vi "HW_6p1_Task1_weesesr.vi"() -> ()   [LabVIEW 2016]
uses:
  <vilib>/express/express arith-compare/Formula/XNode/ExpressFormulaBlockNode.xnode
panel:
  in  "Target Concentration for C (in mol/L)":dbl
  out "Time passed (in min)":dbl
  out "Concentration C":dbl
  out "Concentration B":dbl
  out "Concentration A":dbl
  in  "K3 (in mol^4/min)":dbl
  in  "K2 (in L / mol*min)":dbl
  in  "K1 (in L^2 / mol^2 *min)":dbl
  in  "B Initial Concentration":dbl
  in  "A Initial Concentration":dbl
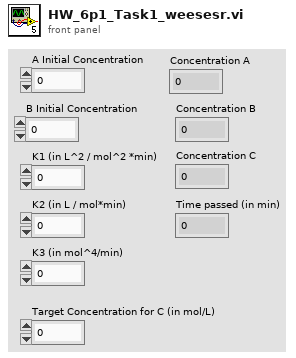
[diagram p1: front panel]
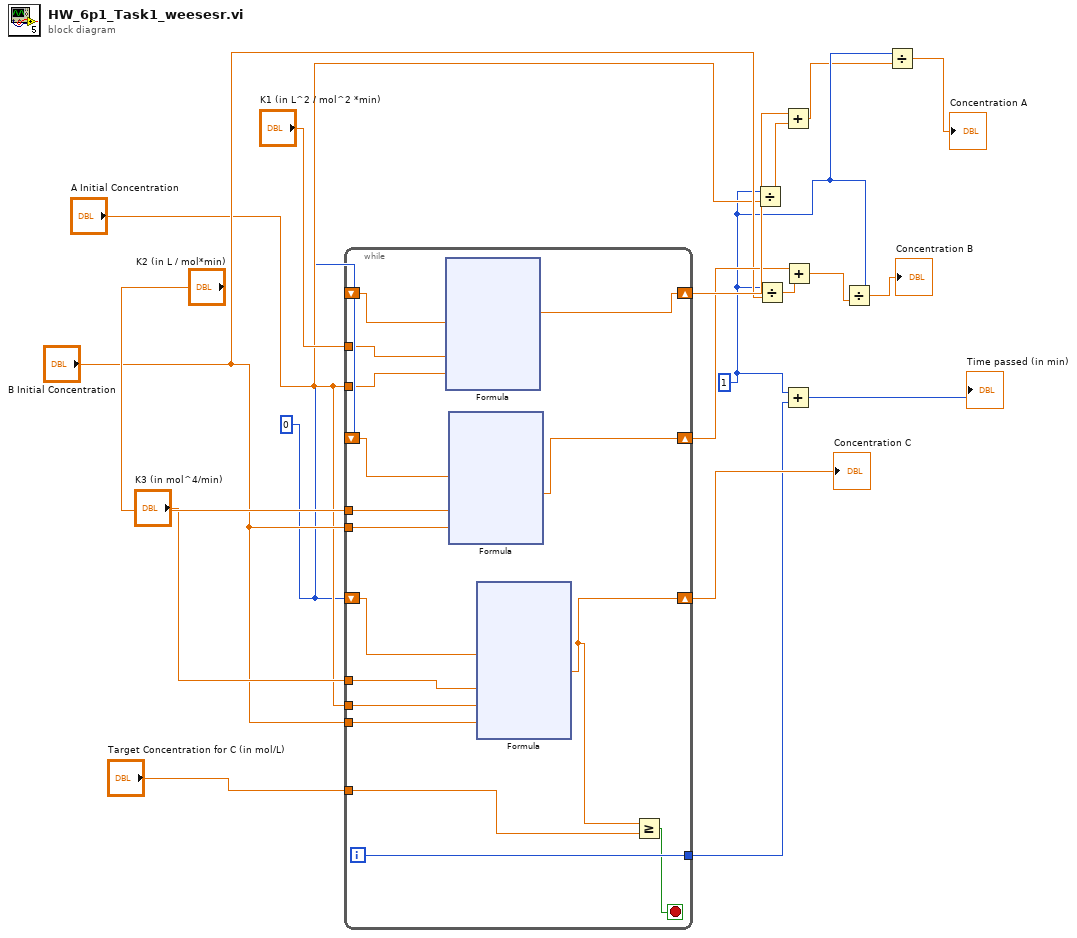
[diagram p0: block diagram]
diagram:
  w8 = 0
  w5 = 1
  n1 = while {
    shift-right: [w20] -> w12
    shift-left: w8 -> [w21]
    tunnel: [w35] -> w7
    shift-right: [w29] -> w11
    shift-left: w8 -> [w30]
    shift-right: [w31] -> w14
    shift-left: w8 -> [w32]
    tunnel: "A Initial Concentration" -> [w34]
    tunnel: "K1 (in L^2 / mol^2 *min)" -> [w33]
    tunnel: "B Initial Concentration" -> [w28]
    tunnel: "K2 (in L / mol*min)" -> [w27]
    tunnel: "K3 (in mol^4/min)" -> [w26]
    tunnel: "Target Concentration for C (in mol/L)" -> [w25]
    tunnel: "B Initial Concentration" -> [w22]
    tunnel: "A Initial Concentration" -> [w23]
    i -> [w35]
    stop <- w24 stop-if-true
    n2 = xnode "Formula"("X1"=w32, "X2"=w33, "X3"=w34) -> ("Result"=w31:dbl)  [unwired: 1 in, 1 out]
    n3 = xnode "Formula"("X1"=w30, "X2"=w27, "X3"=w28) -> ("Result"=w29:dbl)  [unwired: 1 in, 1 out]
    n4 = xnode "Formula"("X1"=w21, "X2"=w26, "X3"=w23, "X4"=w22) -> ("Result"=w20:dbl)  [unwired: 1 in, 1 out]
    n5 = Greater Or Equal?(x=w20, y=w25) -> (x >= y?=w24:bool)
  }
  "Concentration C" <- w12
  n6 = Divide(x=w5, y="A Initial Concentration") -> (x/y=w15:dbl)
  n7 = Divide(x=w5, y="B Initial Concentration") -> (x/y=w13:dbl)
  n8 = Add(x=w14, y=w15) -> (x+y=w4:dbl)
  n9 = Add(x=w5, y=w7) -> (x+y=→"Time passed (in min)":i32)
  n10 = Add(x=w11, y=w13) -> (x+y=w2:dbl)
  n11 = Divide(x=w5, y=w2) -> (x/y=→"Concentration B":dbl)
  n12 = Divide(x=w5, y=w4) -> (x/y=→"Concentration A":dbl)
